vi "get time.vi"(10 "item count":dbl, 11 "input_array_time":string[](array[string])) -> (3 "midVar_time":string[](array[string]))   [LabVIEW 2011]
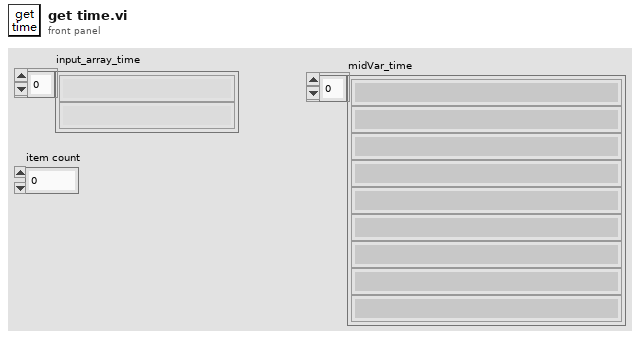
[diagram p1: front panel]
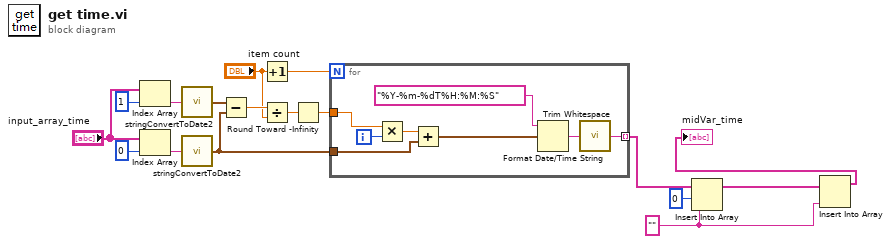
[diagram p0: block diagram]
diagram:
  w2 = "" ("新元素/子数组")
  n1 = Index Array(array="input_array_time", index=1 ("索引")) -> (element=w11:string)
  n2 = Index Array(array="input_array_time", index=0 ("索引")) -> (element=w12:string)
  n3 = call "stringConvertToDate2.vi"("input_str_yymmdd"=w11) -> ("show_date"=w13:timestamp)
  n4 = call "stringConvertToDate2.vi"("input_str_yymmdd"=w12) -> ("show_date"=w17:timestamp)
  n5 = Subtract(x=w13, y=w17) -> (x-y=w14:dbl)
  n6 = Increment(x="item count") -> (x+1=w6:dbl)
  n7 = Divide(x=w14, y="item count") -> (x/y=w15:dbl)
  n8 = Round Toward -Infinity(1:w15) -> (0:w16:dbl)
  n9 = for {
    N: w6 -> [_]
    tunnel: w16 -> [w25]
    tunnel: w17 -> [w23]
    tunnel: [w18] -> w5 mode=indexing
    i -> [w24]
    n10 = Multiply(x=w25, y=w24) -> (x*y=w22:dbl)
    n11 = Add(x=w22, y=w23) -> (x+y=w19:timestamp)
    n12 = Format Date/Time String(time format string (%c)="%Y-%m-%dT%H:%M:%S" ("时间格式字符串(%c)"), seconds (now)=w19) -> (date/time string=w20:string)  [unwired: 1 in]
    n13 = call <vilib>:"Trim Whitespace.vi"("string"=w20) -> ("trimmed string"=w18:string)  [unwired: 1 in]
  }
  n14 = Insert Into Array(array=w5, index=0 ("索引"), new element=w2) -> (w3:string[])
  n15 = Insert Into Array(array=w3, new element=w2) -> (→"midVar_time":string[])  [unwired: 1 in]
